vi "PresetHeight.vi"(11 "Cluster":T1={"Drive Forward Input "=0.0, "Drive Twist Input"=0.0, "Drive Output"=0.05001255502511005, "Drivetwist Output"=0.0, "Left Joystick Buttons"=[FALSE, FALSE, FALSE, FALSE, FALSE, FALSE, FALSE, FALSE, FALSE, FALSE, FALSE, FALSE], "Left Joystick Axis"=[-0.047244094488188976, 0.007874015748031496, -0.0, 1.0], "Right Joystick Axis"=[-0.007874015748031496, -0.007874015748031496, 0.0, -0.4409448818897638], "Right Joystick Button"=[FALSE, FALSE, FALSE, FALSE, FALSE, FALSE, FALSE, FALSE, FALSE, FALSE, FALSE, FALSE], "Arm Encoder"=977.0, "Left Drive Encoder"=-12996.0, "Right Drive Encoder"=21571.0, "Gyro Angle "=0.0, "Arm Joystick Output  "=0.0, "Line Follower L, C, R "=[TRUE, TRUE, TRUE], "Line follow?"=FALSE, " Climb Solenoid"=FALSE, "Wrist Encoder Count"=-55.0, "Wrist Joystick Output"=0.0, "Ball Encoder Count"=0.0, "Ball Output"=0.0, "Climb Encoder"=0.0, "Climb Motor Output"=0.0, " Hatch Solenoid"=FALSE, "Arm Setpoint "=0.0, "Wrist Setpoint "=0.0, "Arm Joystick Enabled?"=FALSE, "Wrist Joystick Enabled"=FALSE, "Vision String"="", "Left Joystick POVs"=[]}) -> (3 "Numeric":dbl format="%#_13g")   [LabVIEW 2018]
uses:
  TypeDefs/Teleop Data Cluster.ctl
  TypeDefs/Joystick Buttons.ctl
panel:
  in  "Lookup Table":dbl[](array[numeric])=[0.0, 1.0, 2.0, 3.0, 4.0, 5.0, 6.0]
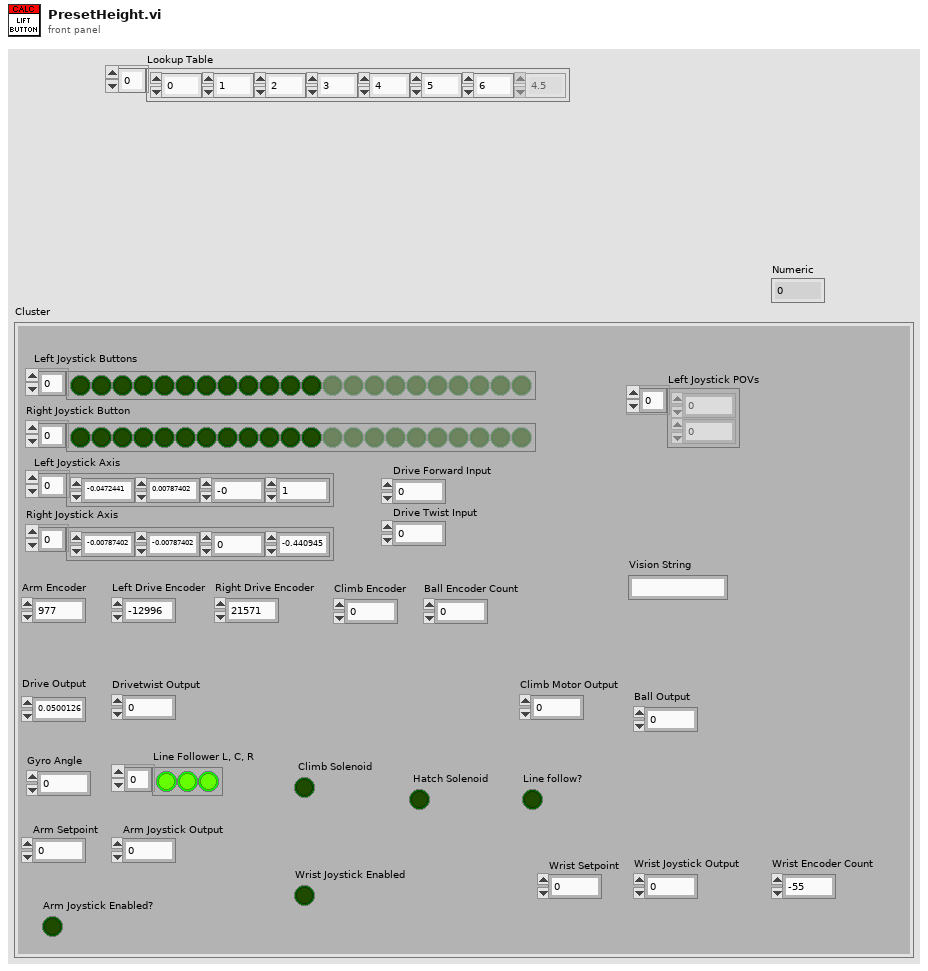
[diagram p1: front panel]
types:
  T1 = typedef "Teleop Data Cluster.ctl" = cluster{"Drive Forward Input ":dbl, "Drive Twist Input":dbl, "Drive Output":dbl, "Drivetwist Output":dbl, "Left Joystick Buttons":bool[], "Left Joystick Axis":dbl[], "Right Joystick Axis":dbl[], "Right Joystick Button":bool[], "Arm Encoder":dbl, "Left Drive Encoder":dbl, "Right Drive Encoder":dbl, "Gyro Angle ":dbl, "Arm Joystick Output  ":dbl, "Line Follower L, C, R ":bool[], "Line follow?":bool, " Climb Solenoid":bool, "Wrist Encoder Count":dbl, "Wrist Joystick Output":dbl, "Ball Encoder Count":dbl, "Ball Output":dbl, "Climb Encoder":dbl, "Climb Motor Output":dbl, " Hatch Solenoid":bool, "Arm Setpoint ":dbl, "Wrist Setpoint ":dbl, "Arm Joystick Enabled?":bool, "Wrist Joystick Enabled":bool, "Vision String":string, "Left Joystick POVs":i16[]}
  T2 = typedef "Joystick Buttons.ctl" = enum16{"Trigger", "Thumb", "Top 3", "Top 4", "Top 5", "Top 6", "Bottom 7", "Bottom 8", "Bottom 9", "Bottom 10", "Bottom 11", "Bottom 12"}
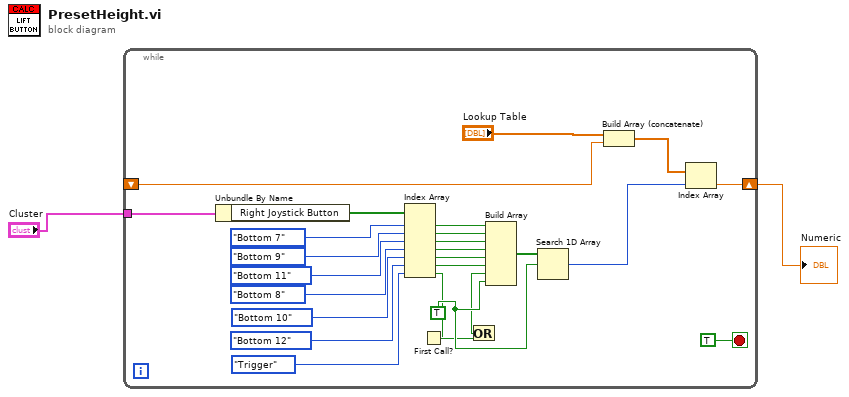
[diagram p0: block diagram]
diagram:
  n1 = while {
    shift-right: [w15] -> w2
    shift-left: _ -> [w13]
    tunnel: "Cluster" -> [w12]
    stop <- TRUE stop-if-true
    w6 = TRUE ("element")
    n2 = Unbundle By Name(w12) -> ("Right Joystick Button"=w28:bool[])
    n3 = Index Array(array=w28, index #1=Joystick_Buttons."Bottom 7" ("Enum"), index #2=Joystick_Buttons."Bottom 9" ("Enum"), index #3=Joystick_Buttons."Bottom 11" ("Enum"), index #4=Joystick_Buttons."Bottom 8" ("Enum"), index #5=Joystick_Buttons."Bottom 10" ("Enum"), index #6=Joystick_Buttons."Bottom 12" ("Enum"), index #7=Joystick_Buttons."Trigger" ("Enum")) -> (element #1=w23:bool, element #2=w22:bool, element #3=w21:bool, element #4=w20:bool, element #5=w8:bool, element #6=w7:bool, element #7=w3:bool)
    n4 = First Call?() -> (First Call?: T/F=w4:bool)
    n5 = Or(x=w4, y=w3) -> (x .or. y?=w5:bool)
    n6 = Build Array(w23, w22, w21, w20, w8, w7, w5, w6) -> (w19:bool[])
    n7 = Search 1D Array(1D array=w19, element=w6) -> (index of element=w18:i32)  [unwired: 1 in]
    n8 = Build Array (concatenate)("Lookup Table", w13) -> (w14:dbl[])
    n9 = Index Array(array=w14, index=w18) -> (element=w15:dbl)
  }
  "Numeric" <- w2
